vi "test_push_raster_as_CS.vi"() -> ()   [LabVIEW 2017]
uses:
  <vilib>/Utility/file.llb/Read Delimited Spreadsheet (DBL).vi
panel:
  out "error out":errorcluster
  in  "number-of-pixels":i32=512
  in  "input-path":path=path "Z:/afm-cs/imaging/raster/5microns/parents/raster_scan_512pix_5mic_01Hz.csv"
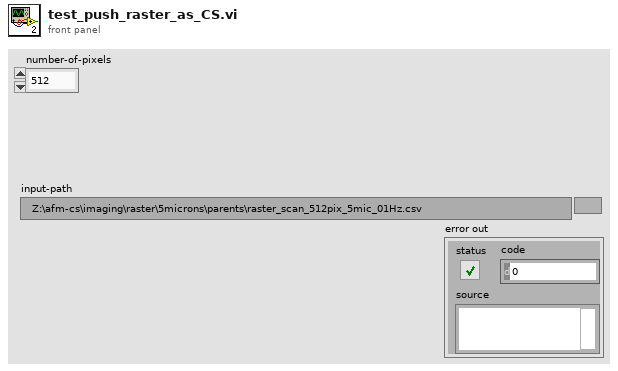
[diagram p1: front panel]
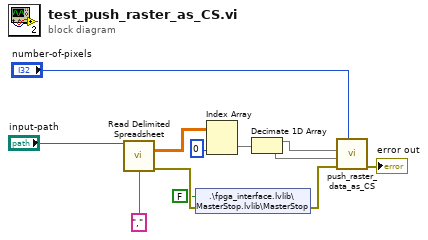
[diagram p0: block diagram]
diagram:
  n1 = call-poly <vilib>:"Read Delimited Spreadsheet.vi"("file path (dialog if empty)"="input-path", "delimiter (\\t)"=",") -> ("all rows"=w10:dbl[][], "error out"=w3:errorcluster)  [unwired: 8 in, 4 out]
  n2 = shared-variable ".\\fpga_interface.lvlib\\MasterStop.lvlib\\MasterStop"(FALSE ("MasterStop"), error in=w3) -> (error out=w2:errorcluster)
  n3 = Index Array(array=w10, index (col)=0 ("dimension size")) -> (element=w8:dbl[])  [unwired: 1 in]
  n4 = Decimate 1D Array(w8) -> (w7:dbl[], w6:dbl[])
  n5 = call "push_raster_data_as_CS.vi"("number-of-pixels"="number-of-pixels", "error in"=w2, "base y_ref (ramp)"=w6, "base x_ref(triangle wave)"=w7) -> ("error out"=→"error out":errorcluster)  [unwired: 6 in, 1 out]
